vi "DriveControl.vi"(9 "Buttons":bool[](array[boolean]), 10 "Axes":dbl[](array[numeric]), 11 "RobotDriveDevRef":T1={"DevStatus"={"status"=FALSE, "code"=0, "source"=""}, "Motors[]"=[], "Square Inputs"=FALSE, "Max Output"=1.0}) -> (2 "Motor Values":dbl[](array[numeric]))   [LabVIEW 2015]
uses:
  <vilib>/Rock Robotics/WPI/RobotDrive/WPI_RobotDriveDevRef.ctl
  <vilib>/Rock Robotics/WPI/MotorControl/WPI_MotorControlDeviceRef.ctl
  <vilib>/Rock Robotics/WPI/MotorControl/WPI_MotorControlType.ctl
  <vilib>/Rock Robotics/SystemInterfaces/DIO/FPGA_DIOPWMChannel.ctl
  <vilib>/Rock Robotics/WPI/PWM/WPI_PWMDeadband.ctl
  <vilib>/Rock Robotics/WPI/CAN/Jaguar/SubVIs/WPI_CANJaguar_ControlMode.ctl
  <vilib>/Rock Robotics/WPI/CAN/TalonSRX/WPI_CANTalonSRX_APIControlMode.ctl
  <vilib>/Rock Robotics/Network Tables/NT Read Number.vi
panel:
  in  "error in (no error)":errorcluster
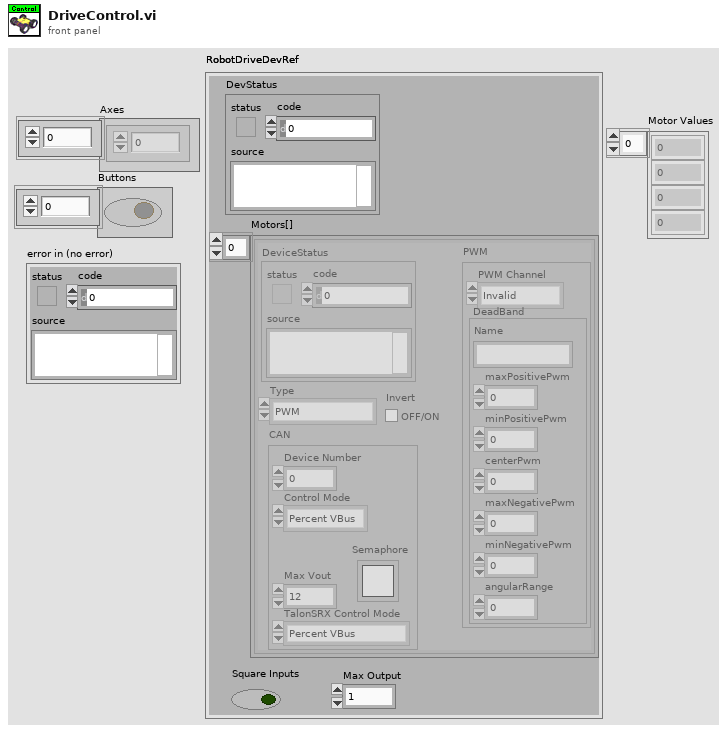
[diagram p1: front panel]
types:
  T1 = typedef "WPI_RobotDriveDevRef.ctl" = cluster{"DevStatus":errorcluster, "Motors[]":T2[], "Square Inputs":bool, "Max Output":dbl}
  T2 = typedef "WPI_MotorControlDeviceRef.ctl" = cluster{"DeviceStatus":errorcluster, "Type":T3, "PWM":cluster{"PWM Channel":T4, "DeadBand":T5}, "CAN":cluster{"Device Number":u8, "Control Mode":T6, "Semaphore":T7, "Max Vout":dbl, "TalonSRX Control Mode":T8}, "Invert":bool}
  T3 = typedef "WPI_MotorControlType.ctl" = enum16{"PWM", "CAN", "CANTalonSRX"}
  T4 = typedef "FPGA_DIOPWMChannel.ctl" = enum8{"PWM 0", "PWM 1", "PWM 2", "PWM 3", "PWM 4", "PWM 5", "PWM 6", "PWM 7", "PWM 8", "PWM 9", "PWM MXP 0", "PWM MXP 1", "PWM MXP 2", "PWM MXP 3", "PWM MXP 4", "PWM MXP 5", "PWM MXP 6", "PWM MXP 7", "PWM MXP 8", "PWM MXP 9", "Invalid"}
  T5 = typedef "WPI_PWMDeadband.ctl" = cluster{"Name":string, "maxPositivePwm":i32, "minPositivePwm":i32, "centerPwm":i32, "maxNegativePwm":i32, "minNegativePwm":i32, "angularRange":u16}
  T6 = typedef "WPI_CANJaguar_ControlMode.ctl" = enum8{"Percent VBus", "Current", "Speed", "Position", "Voltage"}
  T7 = typedef "Semaphore RefNum" = refnum<k1>
  T8 = typedef "WPI_CANTalonSRX_APIControlMode.ctl" = enum8{"Percent VBus", "Speed", "Position", "Slave", "Unchanged / Invalid", "Voltage Compensation", "Current", "Motion Profile"}
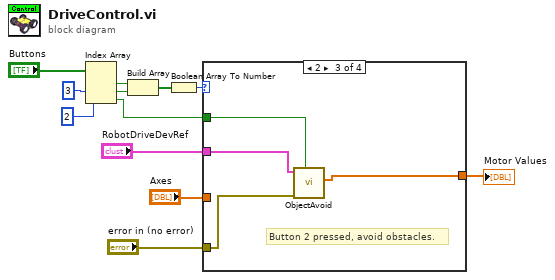
[diagram p0: block diagram]
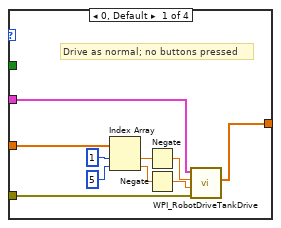
[diagram p2: hidden frame]
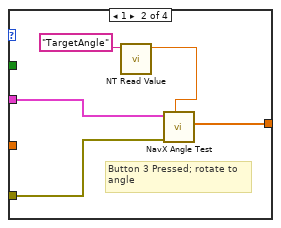
[diagram p3: hidden frame]
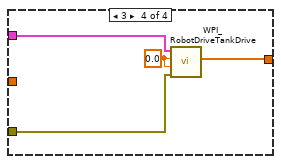
[diagram p4: hidden frame]
diagram:
  n1 = Index Array(array="Buttons", index #2=3 ("index"), index #3=2 ("index")) -> (element #1=w9:bool, element #2=w8:bool, element #3=w1:bool)  [unwired: 1 in]
  n2 = Build Array(w9, w8) -> (w7:bool[])
  n3 = Boolean Array To Number(Boolean array=w7) -> (number=w6:u32)
  n4 = case shown="2" w6 {
    tunnel: "Axes" -> [w20 _ _ _]
    tunnel: "RobotDriveDevRef" -> [w15 w27 w31 w34]
    tunnel: "error in (no error)" -> [w14 w26 w30 w33]
    tunnel: [w13 w23 w29 w35] -> w3
    tunnel: w1 -> [_ _ w28 _]
    frame 0, Default {
      # "Drive as normal; no buttons pressed"
      n5 = Index Array(array=w20, index #1=1 ("index"), index #2=5 ("index")) -> (element #1=w22:dbl, element #2=w21:dbl)
      n6 = Negate(x=w22) -> (-x=w17:dbl)
      n7 = Negate(x=w21) -> (-x=w16:dbl)
      n8 = call <vilib>:"WPI_RobotDriveTankDrive.vi"("error in (no error)"=w14, "Right axis value"=w16, "Left axis value"=w17, "RobotDriveDevRef"=w15) -> ("Motor Values"=w13:dbl[])  [unwired: 5 in, 2 out]
    }
    frame 1 {
      # "Button 3 Pressed; rotate to \nangle"
      n9 = call-poly <vilib>:"NT Read Value.vi"("Name"="TargetAngle") -> ("Numeric"=w24:dbl)  [unwired: 9 in, 1 out]
      n10 = call "NavX Angle Test.vi"("Target Angle"=w24, "Error In"=w26, "RobotDriveDevRefnum"=w27) -> ("Motor Values"=w23:dbl[])  [unwired: 6 in, 2 out]
    }
    frame 2 {
      # "Button 2 pressed, avoid obstacles."
      n11 = call "ObjectAvoid.vi"("Stop?"=w28, "error in (no error)"=w30, "RobotDriveDevRef"=w31) -> ("Motor Values"=w29:dbl[])  [unwired: 8 in]
    }
    frame 3 {
      w32 = 0.0 ("Left axis value")
      n12 = call <vilib>:"WPI_RobotDriveTankDrive.vi"("error in (no error)"=w33, "Right axis value"=w32, "Left axis value"=w32, "RobotDriveDevRef"=w34) -> ("Motor Values"=w35:dbl[])  [unwired: 5 in, 2 out]
    }
  }
  "Motor Values" <- w3
